vi "Populate Tree with Delimited Strings_csm.vi"(5 "Use Child Only?":bool, 7 "Default Symbol":i32=37, 8 "error in (no error)":errorcluster, 9 "Delimiter":string=".", 10 "Items (Delimited)":string[][](array[string]), 11 "Tree Control":refnum<vi>) -> (0 "error out":errorcluster, 2 "Parents Added":string[](array[string]), 3 "Tree Control Dup":refnum<vi>)   [LabVIEW 2017, in "csm-tool-support.lvlib"]
doc: "Populates the specified Tree Control with the specified items. The items are delimited strings where the text of each parent is in the string seperated by delimiters. For example, the string \"C\\Project\\Foo\" with the delimiter \"\\\" would be shown as\nC\n Project\n Foo\nEach Row in the 2D Items array is a child item. The first column contains the Tags. Subsequent columns contain Text for the Tree control columns.\nIf \"Use Child Only Items?\" is true, then items in the 2D array that are not followed by a descendent item are inserted as \"Child Only\". Otherwise, all items are inserted as Child Only=False. NOTE: If Use Child Only Items? is true, then the 2D array must have all parent tags followed immediately by one child item.\n\nAuthored by Shawn D. Walpole\nsupport@mooregoodideas.com\nwww.mooregoodideas.com\n\nCopyright (c) 2010, Moore Good Ideas, Inc.\n\nAll rights reserved.\n\nRedistribution and use in source and binary forms, with or without modification, are permitted provided that the following conditions are met:\n\n * Redistributions of source code must retain the above copyright notice, this list of conditions and the following disclaimer.\n * Redistributions in binary form must reproduce the above copyright notice, this list of conditions and the following disclaimer in the documentation and/or other materials provided with the distribution.\n * Neither the name of Moore Good Ideas, Inc. nor the names of its contributors may be used to endorse or promote products derived from this software without specific prior written permission.\n\nTHIS SOFTWARE IS PROVIDED BY THE COPYRIGHT HOLDERS AND CONTRIBUTORS \"AS IS\" AND ANY EXPRESS OR IMPLIED WARRANTIES, INCLUDING, BUT NOT LIMITED TO, THE IMPLIED WARRANTIES OF MERCHANTABILITY AND FITNESS FOR A PARTICULAR PURPOSE ARE DISCLAIMED. IN NO EVENT SHALL THE COPYRIGHT OWNER OR CONTRIBUTORS BE LIABLE FOR ANY DIRECT, INDIRECT, INCIDENTAL, SPECIAL, EXEMPLARY, OR CONSEQUENTIAL DAMAGES (INCLUDING, BUT NOT LIMITED TO, PROCUREMENT OF SUBSTITUTE GOODS OR SERVICES; LOSS OF USE, DATA, OR PROFITS; OR BUSINESS INTERRUPTION) HOWEVER CAUSED AND ON ANY THEORY OF LIABILITY, WHETHER IN CONTRACT, STRICT LIABILITY, OR TORT (INCLUDING NEGLIGENCE OR OTHERWISE) ARISING IN ANY WAY OUT OF THE USE OF THIS SOFTWARE, EVEN IF ADVISED OF THE POSSIBILITY OF SUCH DAMAGE."
uses:
  csm-tool-support.lvlib
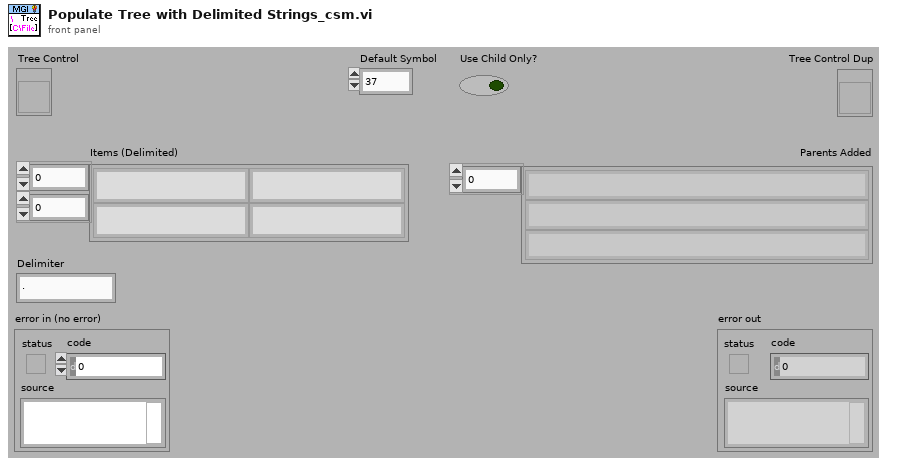
[diagram p1: front panel]
types:
  T1 = cluster{"Left Cell String":string, "Child Text":string[], "Child Tag":string, "Item Indent":i32, "Child Only?":bool, "Glyph Index":i32}[]
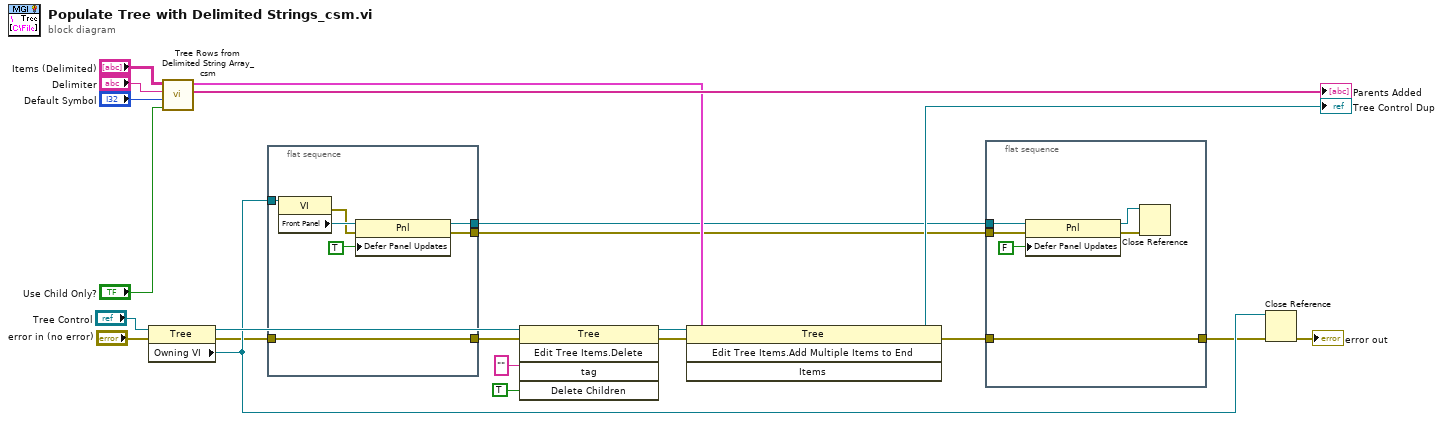
[diagram p0: block diagram]
diagram:
  n1 = property class="Tree"(reference="Tree Control", error in="error in (no error)") -> (reference out=w9:refnum<vi>, error out=w3:errorcluster, "Owning VI"=w7:refnum<vi>)
  n2 = call "Tree Rows from Delimited String Array_csm.vi"("Use Child Only? (F)"="Use Child Only?", "Default Symbol"="Default Symbol", "Delimiter"="Delimiter", "Items (Delimited)"="Items (Delimited)") -> ("Parent Tag Added[]"=→"Parents Added":string[], "Item to Add[]"=w11:T1)  [unwired: 6 in]
  n3 = flat-sequence {
    tunnel: w7 -> [w29]
    tunnel: [w25] -> w6
    tunnel: [w24] -> w5
    tunnel: [w23] -> w4
    tunnel: w3 -> [w23]
    frame #0 {
      n4 = property class="VI"(reference=w29) -> (error out=w26:errorcluster, "Front Panel"=w28:refnum<vi>)  [unwired: 1 in, 1 out]
      n5 = property class="Pnl"(reference=w28, error in=w26, "Defer Panel Updates"=TRUE) -> (reference out=w24:refnum<vi>, error out=w25:errorcluster)
    }
  }
  n6 = invoke on="Invoke Node" class="Tree" method="Edit Tree Items.Delete"(reference=w9, error in=w4, "tag"="" ("Tag"), "Delete Children"=TRUE ("Delete Children?")) -> (reference out=w13:refnum<vi>, error out=w12:errorcluster)  [unwired: 1 in, 3 out]
  n7 = invoke on="Invoke Node" class="Tree" method="Edit Tree Items.Add Multiple Items to End"(reference=w13, error in=w12, "Items"=w11) -> (reference out=→"Tree Control Dup":refnum<vi>, error out=w1:errorcluster)  [unwired: 1 in, 2 out]
  n8 = flat-sequence {
    tunnel: w6 -> [w34]
    tunnel: w5 -> [w33]
    tunnel: [w30] -> w2
    tunnel: w1 -> [w30]
    frame #0 {
      n9 = property class="Pnl"(reference=w33, error in=w34, "Defer Panel Updates"=FALSE) -> (reference out=w31:refnum<vi>, error out=w32:errorcluster)
      n10 = Close Reference(reference=w31, error in (no error)=w32) -> ()  [unwired: 1 out]
    }
  }
  n11 = Close Reference(reference=w7, error in (no error)=w2) -> (error out=→"error out":errorcluster)
